vi "_logging_get_parameter.vi"(5 "Error if not found (T)":bool=TRUE, 7 "Logging Parameter":T1, 8 "error in":errorcluster caption="error in (no error)", 11 "Logging params in":variant) -> (0 "error out":errorcluster, 1 "String parameter out":string, 2 "Int32 parameter out":i32, 3 "Logging params out":variant, 4 "Found":bool)   [LabVIEW 2020, in "Rohde&Schwarz RTx Oscilloscopes.lvlib" / "rsidr_core.lvlib"]
uses:
  rsidr_core.lvlib
  _type_Logging_Parameter.ctl
  type_Error_Codes.ctl
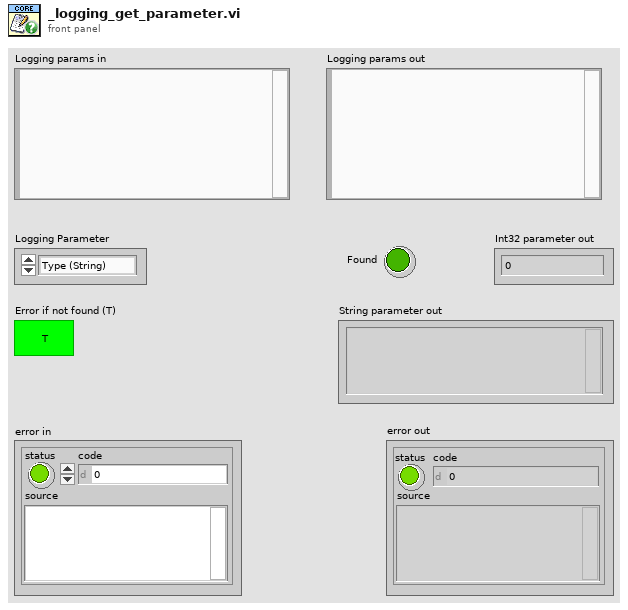
[diagram p1: front panel]
types:
  T1 = typedef "Rohde&Schwarz RTx Oscilloscopes.lvlib/rsidr_core.lvlib/_type_Logging_Parameter.ctl" = enum16{"Type (String)", "SessionAlias(String)", "FormatString (String)", "UDPconectionID (I32)", "UDPlocalPort (I32)", "UDPremotePort (I32)", "UDPremoteHost (String)", "FILEmode (I32)", "FILEpath (String)", "FILEopenID (I32)", "DataMaxLogLen (I32)"}
  T2 = typedef "Rohde&Schwarz RTx Oscilloscopes.lvlib/rsidr_core.lvlib/type_Error_Codes.ctl" = enum16{"No_error", "VISA_err_ResourceNotFound", "VISA_err_Timeout", "VISA_warn_MoreDataAvailable", "RS_err_MissingCallback", "RS_err_InvalidAttribute", "RS_err_InvalidValue", "RS_err_UnknownResource", "RS_err_AlreadyInitialized", "RS_err_InstrumentStatus", "RS_err_BadRepCapName", "RS_err_TypesMismatch", "RS_err_ValueNotSupported", "RS_err_InvalidRngTable", "RS_err_IDqueryFail", "RS_err_UnexpResponse", "VISA_warn_ConfigNotLoaded", "RS_err_AttributeNotReadable", "RS_err_AttributeNotWritable", "RS_err_InstrumentType", "RS_err_InstrumentOption", "VISA_err_InvalidSize", "RS_err_ReliabilityIndicator", "VISA_warn_UnknownStatus", "VISA_warn_TermCharRead", "VISA_err_IO_error", "RS_err_FunctionNotSupported", "VISA_warn_QueueEmpty"}
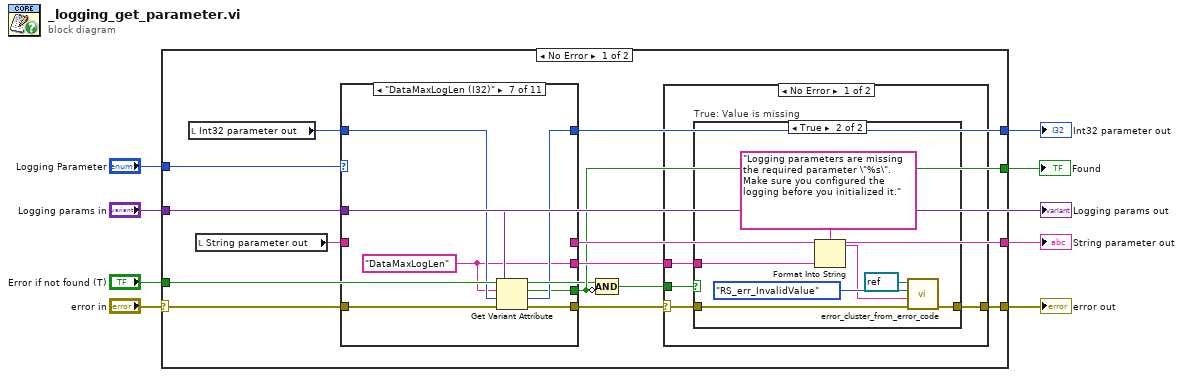
[diagram p0: block diagram]
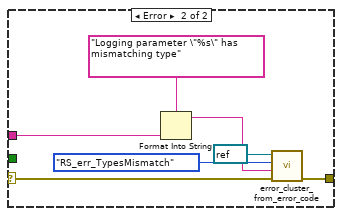
[diagram p3: hidden frame]
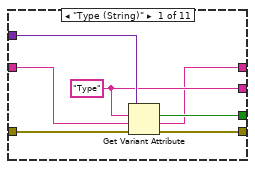
[diagram p4: hidden frame]
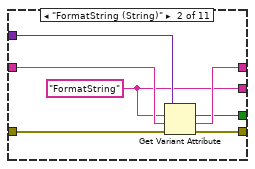
[diagram p5: hidden frame]
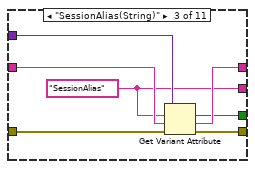
[diagram p6: hidden frame]
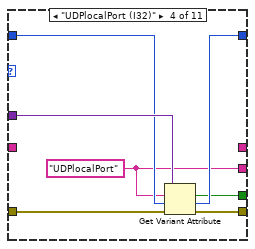
[diagram p7: hidden frame]
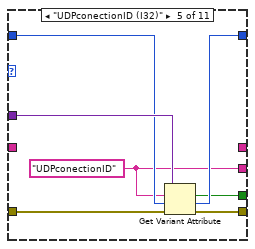
[diagram p8: hidden frame]
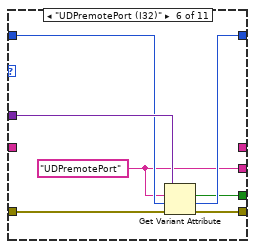
[diagram p9: hidden frame]
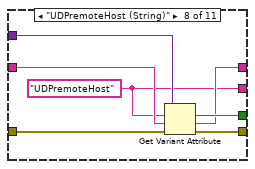
[diagram p10: hidden frame]
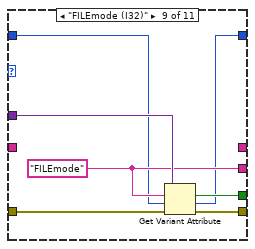
[diagram p11: hidden frame]
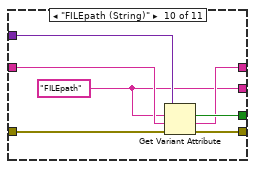
[diagram p12: hidden frame]
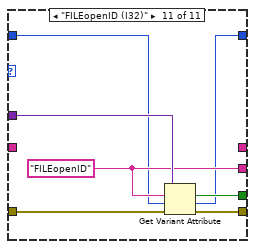
[diagram p13: hidden frame]
diagram:
  n1 = case shown="No Error" "error in" {
    selector: "error in" -> [w21 w118]
    tunnel: [w14 w118] -> w7
    tunnel: "Logging params in" -> [w20 _]
    tunnel: [w18 _] -> w6
    tunnel: [w17 _] -> w5
    tunnel: [w11 _] -> w3
    tunnel: "Error if not found (T)" -> [w10 _]
    tunnel: "Logging Parameter" -> [w9 _]
    frame No Error {
      n2 = local read "Int32 parameter out"() -> (w19:i32)
      n3 = local read "String parameter out"() -> (w16:string)
      n4 = case shown="\"DataMaxLogLen (I32)\"" w9 {
        tunnel: w21 -> [w47 w54 w61 w68 w75 w82 w89 w96 w103 w110 w117]
        tunnel: [w46 w53 w60 w67 w74 w81 w88 w95 w102 w109 w116] -> w15
        tunnel: w20 -> [w45 w52 w59 w66 w73 w80 w87 w94 w101 w108 w115]
        tunnel: w19 -> [_ _ _ w65 w72 w79 w86 _ w97 _ w111]
        tunnel: w16 -> [w42 w51 w58 _ _ _ _ w93 _ w107 _]
        tunnel: [w41 w50 w57 _ _ _ _ w91 _ w105 _] -> w18
        tunnel: [_ _ _ w64 w71 w78 w85 _ w98 _ w112] -> w17
        tunnel: [w44 w49 w56 w63 w70 w77 w84 w92 w100 w106 w114] -> w11
        tunnel: [w43 w48 w55 w62 w69 w76 w83 w90 w99 w104 w113] -> w13
        frame "Type (String)" {
          w43 = "Type"
          n5 = Get Variant Attribute(Variant=w45, name=w43, default value (empty Variant)=w42, error in=w47) -> (found=w44:bool, value=w41:string, error out=w46:errorcluster)  [unwired: 1 out]
        }
        frame "FormatString (String)" {
          w48 = "FormatString"
          n6 = Get Variant Attribute(Variant=w52, name=w48, default value (empty Variant)=w51, error in=w54) -> (found=w49:bool, value=w50:string, error out=w53:errorcluster)  [unwired: 1 out]
        }
        frame "SessionAlias(String)" {
          w55 = "SessionAlias"
          n7 = Get Variant Attribute(Variant=w59, name=w55, default value (empty Variant)=w58, error in=w61) -> (found=w56:bool, value=w57:string, error out=w60:errorcluster)  [unwired: 1 out]
        }
        frame "UDPlocalPort (I32)" {
          w62 = "UDPlocalPort"
          n8 = Get Variant Attribute(Variant=w66, name=w62, default value (empty Variant)=w65, error in=w68) -> (found=w63:bool, value=w64:i32, error out=w67:errorcluster)  [unwired: 1 out]
        }
        frame "UDPconectionID (I32)" {
          w69 = "UDPconectionID"
          n9 = Get Variant Attribute(Variant=w73, name=w69, default value (empty Variant)=w72, error in=w75) -> (found=w70:bool, value=w71:i32, error out=w74:errorcluster)  [unwired: 1 out]
        }
        frame "UDPremotePort (I32)" {
          w76 = "UDPremotePort"
          n10 = Get Variant Attribute(Variant=w80, name=w76, default value (empty Variant)=w79, error in=w82) -> (found=w77:bool, value=w78:i32, error out=w81:errorcluster)  [unwired: 1 out]
        }
        frame "DataMaxLogLen (I32)" {
          w83 = "DataMaxLogLen"
          n11 = Get Variant Attribute(Variant=w87, name=w83, default value (empty Variant)=w86, error in=w89) -> (found=w84:bool, value=w85:i32, error out=w88:errorcluster)  [unwired: 1 out]
        }
        frame "UDPremoteHost (String)" {
          w90 = "UDPremoteHost"
          n12 = Get Variant Attribute(Variant=w94, name=w90, default value (empty Variant)=w93, error in=w96) -> (found=w92:bool, value=w91:string, error out=w95:errorcluster)  [unwired: 1 out]
        }
        frame "FILEmode (I32)" {
          w99 = "FILEmode"
          n13 = Get Variant Attribute(Variant=w101, name=w99, default value (empty Variant)=w97, error in=w103) -> (found=w100:bool, value=w98:i32, error out=w102:errorcluster)  [unwired: 1 out]
        }
        frame "FILEpath (String)" {
          w104 = "FILEpath"
          n14 = Get Variant Attribute(Variant=w108, name=w104, default value (empty Variant)=w107, error in=w110) -> (found=w106:bool, value=w105:string, error out=w109:errorcluster)  [unwired: 1 out]
        }
        frame "FILEopenID (I32)" {
          w113 = "FILEopenID"
          n15 = Get Variant Attribute(Variant=w115, name=w113, default value (empty Variant)=w111, error in=w117) -> (found=w114:bool, value=w112:i32, error out=w116:errorcluster)  [unwired: 1 out]
        }
      }
      n16 = Compound Arithmetic op=AND(w10, invert w11) -> (w12:bool)
      n17 = case shown="No Error" w15 {
        selector: w15 -> [w23 w39]
        tunnel: [w25 w40] -> w14
        tunnel: w13 -> [w24 w38]
        tunnel: w12 -> [w22 _]
        frame No Error {
          n18 = case "True: Value is missing" shown="True" w22 {
            tunnel: w23 -> [w26 w30]
            tunnel: [w26 w33] -> w25
            tunnel: w24 -> [_ w31]
            frame False {
            }
            frame True {
              n19 = Format Into String(format string="Logging parameters are missing the required parameter \"%s\". Make sure you configured the logging before you initialized it.", w31) -> (resulting string=w28:string)  [unwired: 2 in, 1 out]
              n20 = call "error_cluster_from_error_code.vi"("error in"=w30, "Error Message (\"\")"=w28, "Error Enum in"=type_Error_Codes."RS_err_InvalidValue", "VISA resource name"=refnum<visa-resource-name> refnum) -> ("error out"=w33:errorcluster)  [unwired: 6 in, 1 out]
            }
          }
        }
        frame Error {
          n21 = Format Into String(format string="Logging parameter \"%s\" has mismatching type", w38) -> (resulting string=w35:string)  [unwired: 2 in, 1 out]
          n22 = call "error_cluster_from_error_code.vi"("error in"=w39, "Error Message (\"\")"=w35, "Error Enum in"=type_Error_Codes."RS_err_TypesMismatch", "VISA resource name"=refnum<visa-resource-name> refnum) -> ("error out"=w40:errorcluster)  [unwired: 6 in, 1 out]
        }
      }
    }
    frame Error {
    }
  }
  "error out" <- w7
  "Int32 parameter out" <- w5
  "String parameter out" <- w6
  "Found" <- w3
  "Logging params out" <- "Logging params in"
